vi "Set Display Ref.vi"(8 "error in (no error)":errorcluster, 10 "Display Ref":refnum<vi>, 11 "Handler.UserEvent.Console in":refnum<class "Handler.UserEvent.Console.lvclass">) -> (0 "error out":errorcluster, 3 "Handler.UserEvent.Console out":refnum<class "Handler.UserEvent.Console.lvclass">)   [LabVIEW 2017, in "Error Log.lvlib" / "Handler.UserEvent.Console.lvclass"]
uses:
  Handler.UserEvent.Console.lvclass
  Handler.UserEvent.Console.lvclass/Handler.UserEvent.Console.ctl
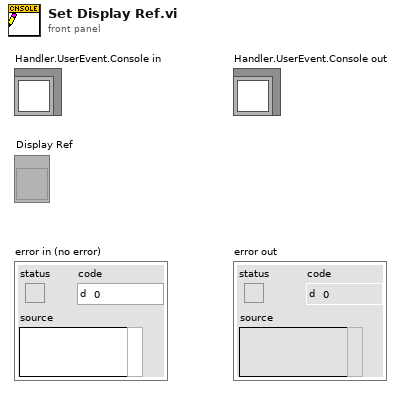
[diagram p1: front panel]
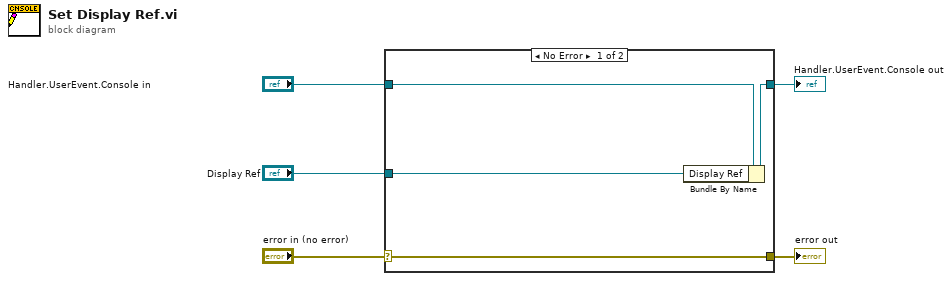
[diagram p0: block diagram]
diagram:
  n1 = case shown="No Error" "error in (no error)" {
    selector: "error in (no error)" -> [w9 w10]
    tunnel: [w9 w10] -> w4
    tunnel: [w7 w11] -> w2
    tunnel: "Handler.UserEvent.Console in" -> [w8 w11]
    tunnel: "Display Ref" -> [w6 _]
    frame No Error {
      n2 = Bundle By Name(cluster=w8, "Display Ref"=w6) -> (w7:refnum<class "Handler.UserEvent.Console.lvclass">)
    }
    frame Error {
    }
  }
  "error out" <- w4
  "Handler.UserEvent.Console out" <- w2
